vi "Read PWM Length.vi"(8 "error in (no error)":errorcluster, 11 "Set Length Msg in":refnum<class "Set Length Msg.lvclass">) -> (0 "error out":errorcluster, 2 "PWM Length":dbl[unit]=1.0 format="%.1g", 3 "Set Length Msg out":refnum<class "Set Length Msg.lvclass">)   [LabVIEW 2017, in "BNT_DAQmx.lvlib" / "Set Length Msg.lvclass"]
uses:
  Set Length Msg.lvclass
  Set Length Msg.lvclass/Set Length Msg.ctl
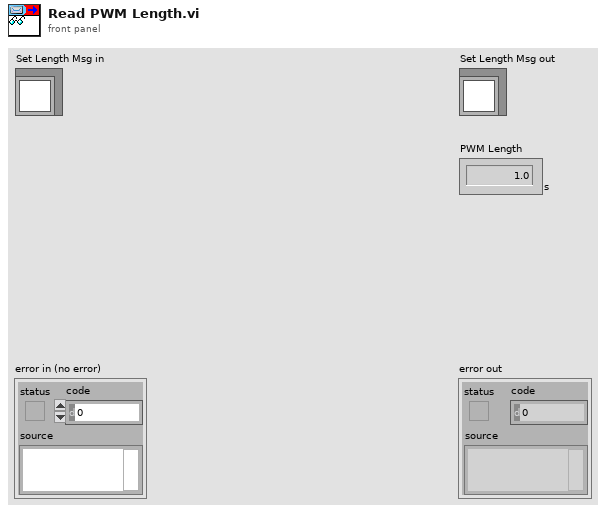
[diagram p1: front panel]
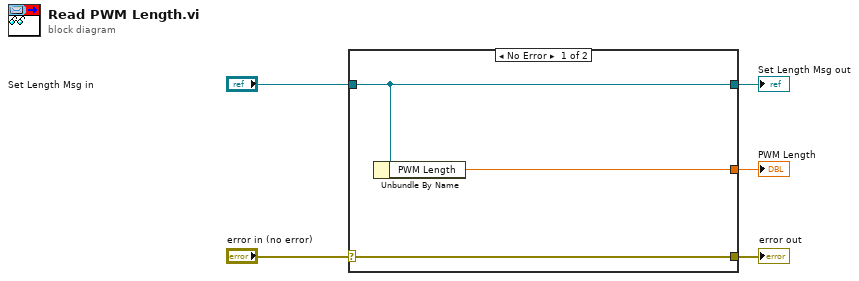
[diagram p0: block diagram]
diagram:
  n1 = case shown="No Error" "error in (no error)" {
    selector: "error in (no error)" -> [w8 w9]
    tunnel: [w8 w9] -> w4
    tunnel: [w7 w10] -> w2
    tunnel: "Set Length Msg in" -> [w7 w10]
    tunnel: [w6 _] -> w1
    frame No Error {
      n2 = Unbundle By Name(w7) -> ("PWM Length"=w6:dbl[unit])
    }
    frame Error {
    }
  }
  "error out" <- w4
  "Set Length Msg out" <- w2
  "PWM Length" <- w1
